vi "Send Pre-Addressed Lock Publication.vi"(5 "PublicationPolicy":refnum<class "IPublicationPolicy.lvclass">, 6 "Return Error Transport":refnum<class "ITransport.lvclass">, 7 "Publisher ID":string, 8 "error in (no error)":errorcluster, 9 "Data to Publish":variant, 10 "Datum Name":string, 11 "Lock Publication Msg":refnum<class "Lock Publication Msg.lvclass">) -> (0 "error out":errorcluster)   [LabVIEW 2017, in "IMediator.lvlib" / "Lock Publication Msg.lvclass"]
doc: "Most Actors or VIs that want to publish data will do so with this send VI. Actors who call this method must have been given a pre-addressed Publish Msg prior to the act of sending. (For Actors, this means that they were launched with a pre-addressed Publish Msg or sent one after the Mediator came alive.)\n\n<License>\nCopyright © 2017 Composed Systems, LLC | All rights reserved\nwww.composed.io\n\nAuthor: Ethan Stern <ethan.stern@composed.io>\n\nThis software is provided \"AS IS\" WITHOUT WARRANTIES, either express or implied, AND IS FOR EDUCATIONAL PURPOSES ONLY.\n</License>"
uses:
  Lock Publication Msg.lvclass
  C:/Git/mva-framework/Framework/AbstractMessages/PreAddressedMsg/PreAddressedMsg.lvclass
  C:/Program Files (x86)/National Instruments/LabVIEW 2017/vi.lib/ActorFramework/Message/Message.lvclass
  ITransport/ITransport.lvclass
  IPublicationPolicy/IPublicationPolicy.lvclass
  AbstractMessages/PreAddressedMsg/PreAddressedMsg.lvclass/PreAddressedMsg.ctl
  Lock Publication Msg.lvclass/Lock Publication Msg.ctl
  <vilib>/ActorFramework/Message Enqueuer/Message Enqueuer.lvclass/Message Enqueuer.ctl
  <vilib>/ActorFramework/Message Priority Queue/Priority Enqueue.vi
  <vilib>/ActorFramework/Message Enqueuer/Message Enqueuer.lvclass
  AbstractMessages/PreAddressedMsg/PreAddressedMsg.lvclass
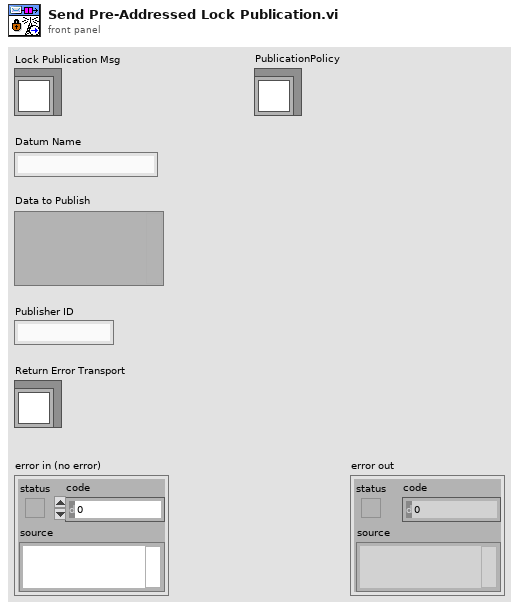
[diagram p1: front panel]
types:
  T1 = typedef "Actor Framework.lvlib/Message Enqueuer.lvclass/Message Priority.ctl" = enum16{"Low", "Normal", "High"}
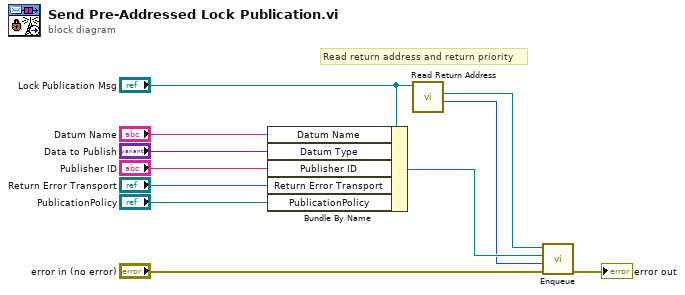
[diagram p0: block diagram]
diagram:
  # "Read return address and return priority"
  n1 = Bundle By Name(cluster="Lock Publication Msg", "Datum Name"="Datum Name", "Datum Type"="Data to Publish", "Publisher ID"="Publisher ID", "Return Error Transport"="Return Error Transport", "PublicationPolicy"="PublicationPolicy") -> (w7:refnum<class "Lock Publication Msg.lvclass">)
  n2 = call "Read Return Address.vi"("PreAddressedMsg in"="Lock Publication Msg") -> ("Return Priority (Normal)"=w4:T1, "Return Address"=w5:refnum<class "Message Enqueuer.lvclass">)  [unwired: 9 in]
  n3 = call <vilib>:"Enqueue.vi"("error in (no error)"="error in (no error)", "Message Priority (Normal)"=w4, "Message"=w7, "Message Enqueuer in"=w5) -> ("error out"=→"error out":errorcluster)  [unwired: 6 in, 1 out]
